vi "SetMeasureRelativeEnable.vi"(7 "Measure Function":T1, 8 "Error In":errorcluster, 9 "Enable?":bool, 10 "SMU":T2, 11 "Keithley 2602 In":refnum<visa-resource-name>) -> (0 "Error Out":errorcluster, 3 "Keithley 2602 Out":refnum<visa-resource-name>)   [LabVIEW 2012, in "Keithley-2602.lvlib"]
uses:
  Keithley-2602.lvlib
  Controls/SMU.ctl
  Controls/MeasureFunction.ctl
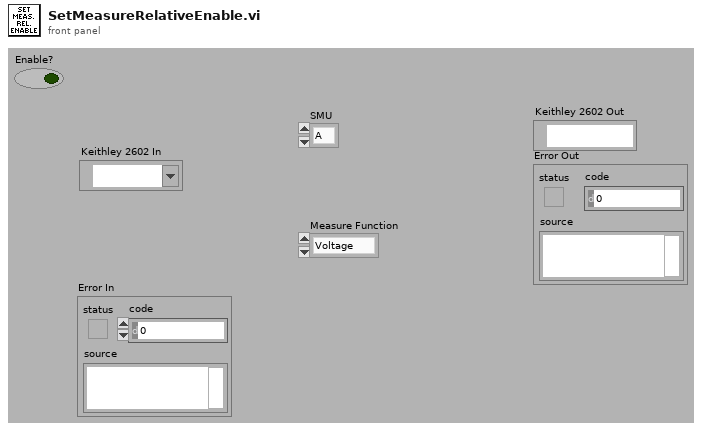
[diagram p1: front panel]
types:
  T1 = typedef "Keithley-2602.lvlib/MeasureFunction.ctl" = enum16{"Voltage", "Current", "Resistance", "Power"}
  T2 = typedef "Keithley-2602.lvlib/SMU.ctl" = enum16{"A", "B"}
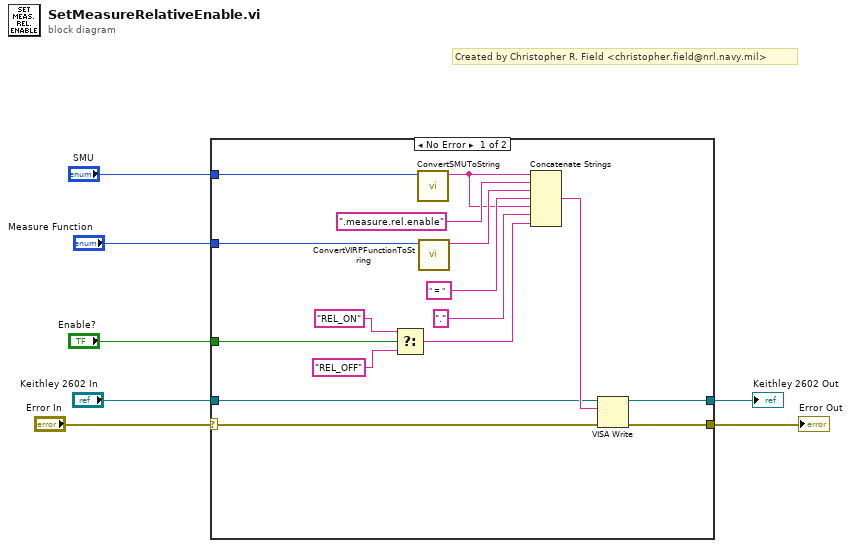
[diagram p0: block diagram]
diagram:
  # "Created by Christopher R. Field <christopher.field@nrl.navy.mil>"
  n1 = case shown="No Error" "Error In" {
    selector: "Error In" -> [w8 w24]
    tunnel: "Keithley 2602 In" -> [w21 w25]
    tunnel: [w20 w25] -> w6
    tunnel: [w19 w24] -> w5
    tunnel: "Enable?" -> [w11 _]
    tunnel: "SMU" -> [w10 _]
    tunnel: "Measure Function" -> [w9 _]
    frame No Error {
      n2 = Select(t="REL_ON", s=w11, f="REL_OFF") -> (s? t:f=w12:string)
      n3 = call "ConvertSMUToString.vi"("SMU"=w10) -> ("Channel"=w16:string)  [unwired: 10 in]
      n4 = call "ConvertVIRPFunctionToString.vi"("Function"=w9) -> ("Function"=w18:string)  [unwired: 10 in]
      n5 = Concatenate Strings(w16, ".measure.rel.enable", w18, " = " ("string"), w16, ".", w12) -> (w22:string)
      n6 = VISA Write(VISA resource name=w21, write buffer=w22, error in (no error)=w8) -> (VISA resource name out=w20:refnum<visa-resource-name>, error out=w19:errorcluster)  [unwired: 1 out]
    }
    frame Error {
    }
  }
  "Keithley 2602 Out" <- w6
  "Error Out" <- w5
